vi "ProjectSilentConnect.vi"(7 "Timeout (60000 ms)":u32=60000, 8 "Calibration File":path, 9 "Undeploy System Definition (F)":bool, 10 "System Definition File (.nivssdf)":path, 11 "Gateway IP Address (\"\": localhost)":string) -> (0 "error out":errorcluster, 3 "ReportText":string)   [LabVIEW 2020, in "ni-veristand-steps-runtime-lib.lvlib"]
uses:
  ni-veristand-steps-runtime-lib.lvlib
  <vilib>/NI VeriStand/Execution/Workspace/NI_VS Workspace ExecutionAPI.lvlib
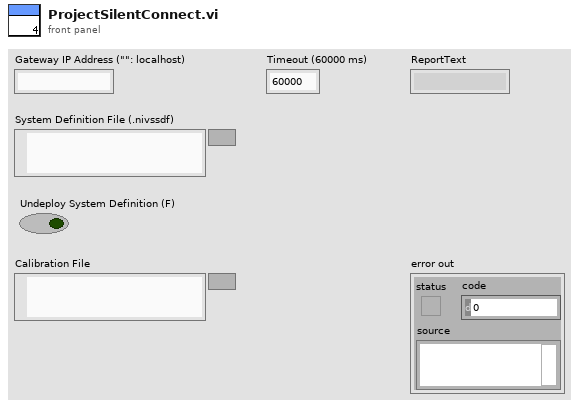
[diagram p1: front panel]
types:
  T1 = typedef "NI_VS Workspace ExecutionAPI.lvlib/WorkspaceAPI.ctl" = refnum<k24>
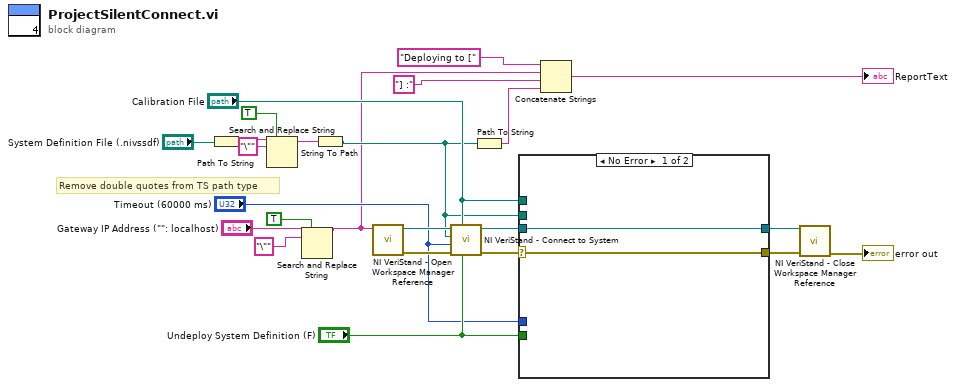
[diagram p0: block diagram]
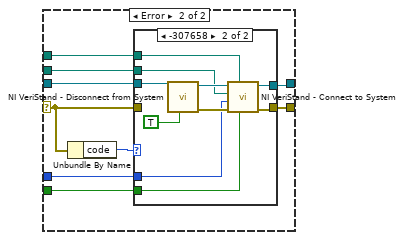
[diagram p2: hidden frame]
diagram:
  # "Remove double quotes from TS path type"
  n1 = Path To String(path="System Definition File (.nivssdf)") -> (string=w16:string)
  n2 = Search and Replace String(replace all?=TRUE ("replace all? (F)"), input string=w16, search string="\"") -> (result string=w14:string)  [unwired: 5 in, 3 out]
  n3 = Search and Replace String(replace all?=TRUE ("replace all? (F)"), input string="Gateway IP Address (\"\": localhost)", search string="\"") -> (result string=w1:string)  [unwired: 5 in, 3 out]
  n4 = String To Path(string=w14) -> (path=w8:path)
  n5 = call <vilib>:"NI VeriStand - Open Workspace Manager Reference.vi"("Gateway IP Address (\"\": localhost)"=w1) -> ("error out"=w24:errorcluster, "WorkspaceManager"=w23:T1)  [unwired: 9 in]
  n6 = call <vilib>:"NI VeriStand - Connect to System.vi"("Deploy System Definition (T)"="Undeploy System Definition (F)", "Calibration File"="Calibration File", "error in (no error)"=w24, "Timeout (60000 ms)"="Timeout (60000 ms)", "System Definition File (.nivssdf)"=w8, "WorkspaceManager in"=w23) -> ("error out"=w6:errorcluster, "WorkspaceManager out"=w11:T1)  [unwired: 4 in]
  n7 = Path To String(path=w8) -> (string=w19:string)
  n8 = case shown="No Error" w6 {
    selector: w6 -> [w26 w34]
    tunnel: [w26 w33] -> w12
    tunnel: w11 -> [w25 w32]
    tunnel: "Undeploy System Definition (F)" -> [_ w31]
    tunnel: "Calibration File" -> [_ w30]
    tunnel: w8 -> [_ w29]
    tunnel: "Timeout (60000 ms)" -> [_ w28]
    tunnel: [w25 w27] -> w5
    frame No Error {
    }
    frame Error {
      n9 = Unbundle By Name(w34) -> ("code"=w35:i32)
      n10 = case shown="-307658" w35 {
        tunnel: w34 -> [w37 _]
        tunnel: [w37 w45] -> w33
        tunnel: w32 -> [w36 w46]
        tunnel: w31 -> [_ w43]
        tunnel: w30 -> [_ w41]
        tunnel: w29 -> [_ w40]
        tunnel: w28 -> [_ w39]
        tunnel: [w36 w38] -> w27
        frame Default {
        }
        frame -307658 {
          n11 = call <vilib>:"NI VeriStand - Disconnect from System.vi"("Undeploy System Definition (F)"=TRUE, "WorkspaceManager in"=w46) -> ("error out"=w44:errorcluster, "WorkspaceManager out"=w42:T1)  [unwired: 8 in]
          n12 = call <vilib>:"NI VeriStand - Connect to System.vi"("Deploy System Definition (T)"=w43, "Calibration File"=w41, "error in (no error)"=w44, "Timeout (60000 ms)"=w39, "System Definition File (.nivssdf)"=w40, "WorkspaceManager in"=w42) -> ("error out"=w45:errorcluster, "WorkspaceManager out"=w38:T1)  [unwired: 4 in]
        }
      }
    }
  }
  n13 = Concatenate Strings("Deploying to [", w1, "] :", w19) -> (→"ReportText":string)
  n14 = call <vilib>:"NI VeriStand - Close Workspace Manager Reference.vi"("error in (no error)"=w12, "WorkspaceManager"=w5) -> ("error out"=→"error out":errorcluster)  [unwired: 9 in]
